vi "Get average spectrum from datafiles (subVi).vi"(2 "error in":errorcluster) -> (0 "error out":errorcluster, 1 "Average array":dbl[][](array[numeric]))   [LabVIEW 2016]
doc: "Calculate the averaged spectrum from the spectra measured by the RGA. The data are read from each file from the directory given in the global variable Config_info, the averaged spectrum is calculated and the files are moved to the \"archives\" subfolder and the averaged spectrum is saved in a \"averaged_spectra\" sub-folder."
uses:
  global/Config_Infos.vi
  <vilib>/Utility/file.llb/Write Delimited Spreadsheet (string).vi
  <vilib>/Utility/file.llb/Write Delimited Spreadsheet (DBL).vi
panel:
  out "concatenated string":string
  in  "spectra_folder_name":string="averaged_spectra"
  in  "archive_folder_name":string="archives"
  out "filenames":string[](array[string])
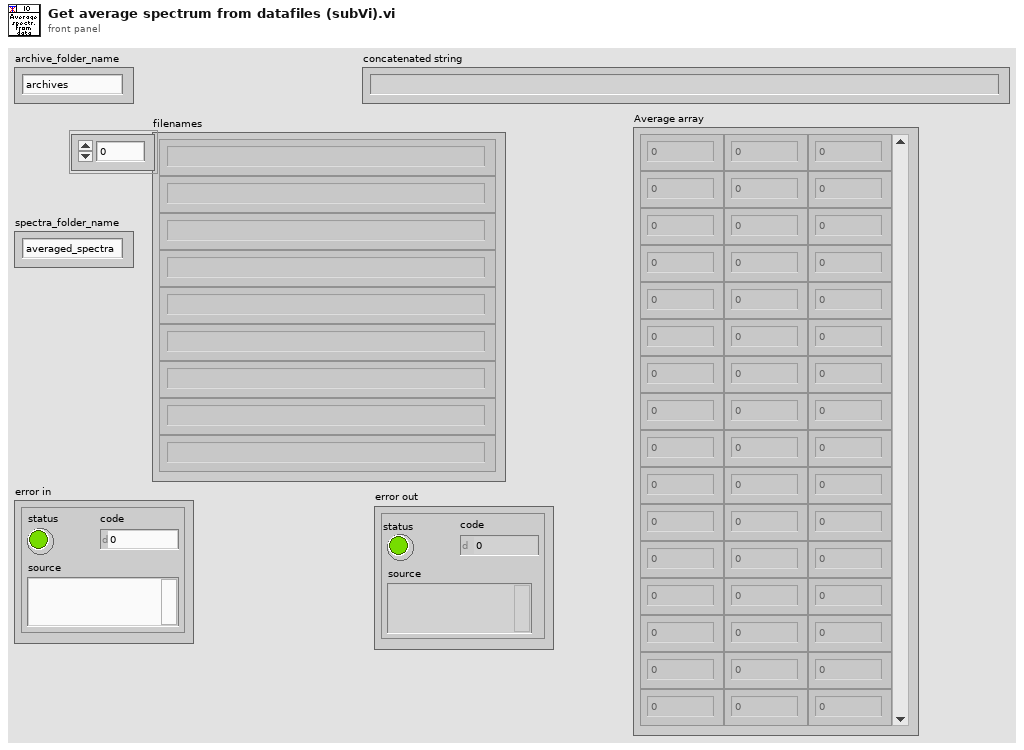
[diagram p1: front panel]
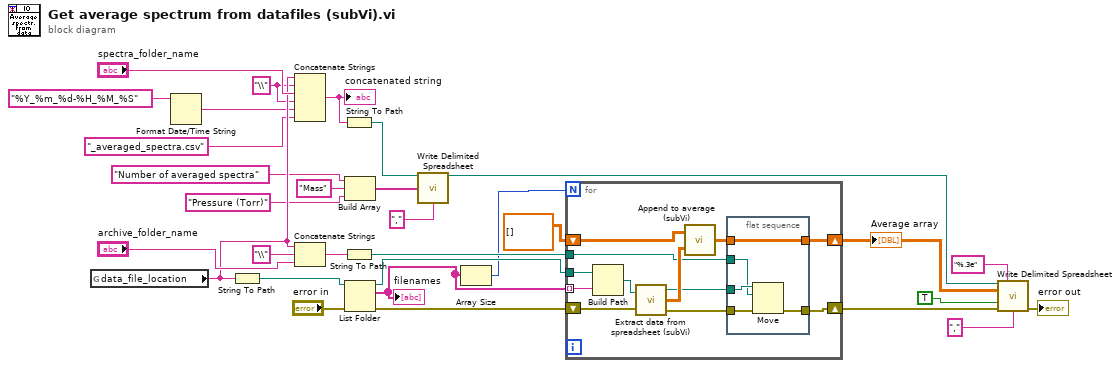
[diagram p0: block diagram]
diagram:
  w17 = "\\" ("string")
  n1 = global read "Config_Infos.vi" "data_file_location"() -> (w19:string)
  n2 = Format Date/Time String(time format string (%c)="%Y_%m_%d-%H_%M_%S") -> (date/time string=w16:string)  [unwired: 2 in]
  n3 = String To Path(string=w19) -> (path=w27:path)
  n4 = Concatenate Strings(w19, w17, "spectra_folder_name", w17, w16, "_averaged_spectra.csv" ("string")) -> (w20:string)
  "concatenated string" <- w20
  n5 = Concatenate Strings(w19, "\\" ("string"), "archive_folder_name") -> (w26:string)
  n6 = String To Path(string=w20) -> (path=w4:path)
  n7 = String To Path(string=w26) -> (path=w25:path)
  n8 = Build Array("Number of averaged spectra", "Mass", "Pressure (Torr)") -> (w5:string[])
  n9 = List Folder(path=w27, error in="error in") -> (path out=w30:path, filenames=w11:string[], error out=w28:errorcluster)  [unwired: 2 in, 1 out]
  "filenames" <- w11
  n10 = call-poly <vilib>:"Write Delimited Spreadsheet.vi"("file path (dialog if empty)"=w4, "1D data"=w5, "delimiter (\\t)"="," ("delimiter (\\t)")) -> ("new file path (Not A Path if cancelled)"=w3:path)  [unwired: 11 in, 1 out]
  n11 = Array Size(array=w11) -> (size(s)=w12:i32)
  n12 = for {
    N: w12 -> [_]
    shift-right: [w37] -> w22
    shift-left: dbl[][] [] ("Average array") -> [w42]
    tunnel: w11 -> [w40] mode=indexing
    tunnel: w30 -> [w41]
    tunnel: w25 -> [w33]
    shift-right: [w32] -> w18
    shift-left: w28 -> [w36]
    n13 = Build Path(base path=w41, name or relative path=w40) -> (appended path=w39:path)
    n14 = call "Extract data from spreadsheet (subVi).vi"("file path (dialog if empty)"=w39, "error in (no error)"=w36) -> ("new file path (Not A Path if cancelled)"=w35:path, "data out"=w43:dbl[][], "error out"=w34:errorcluster)
    n15 = call "Append to average (subVi).vi"("Array in"=w43, "Average array"=w42) -> ("Average array out"=w38:dbl[][])
    n16 = flat-sequence {
      tunnel: w38 -> [w48]
      tunnel: [w48] -> w37
      tunnel: w35 -> [w47]
      tunnel: w34 -> [w46]
      tunnel: w33 -> [w45]
      tunnel: [w44] -> w32
      frame #0 {
        n17 = Move(source path=w47, error in=w46, 10:w45) -> (error out=w44:errorcluster)  [unwired: 2 in, 2 out]
      }
    }
  }
  "Average array" <- w22
  n18 = call-poly <vilib>:"Write Delimited Spreadsheet.vi"("file path (dialog if empty)"=w3, "format (%.3f)"="%.3e", "2D data"=w22, "append to file? (new file:F)"=TRUE, "error in (no error)"=w18, "delimiter (\\t)"="," ("delimiter (\\t)")) -> ("error out"=→"error out":errorcluster)  [unwired: 8 in, 1 out]
